vi "sv_Swept Sine Check for Shift Register.vi"(6 "initialize":bool, 8 "error in (no error)":errorcluster, 9 "elapsed time [s]":dbl format="%.2f") -> (0 "error out":errorcluster, 1 "dup elapsed time [s]":dbl format="%.2f")   [LabVIEW 2017, in "SoundVib_SweptSine.lvlib"]
uses:
  <vilib>/addons/Sound and Vibration/svt_Swept Sine/SoundVib_SweptSine.lvlib
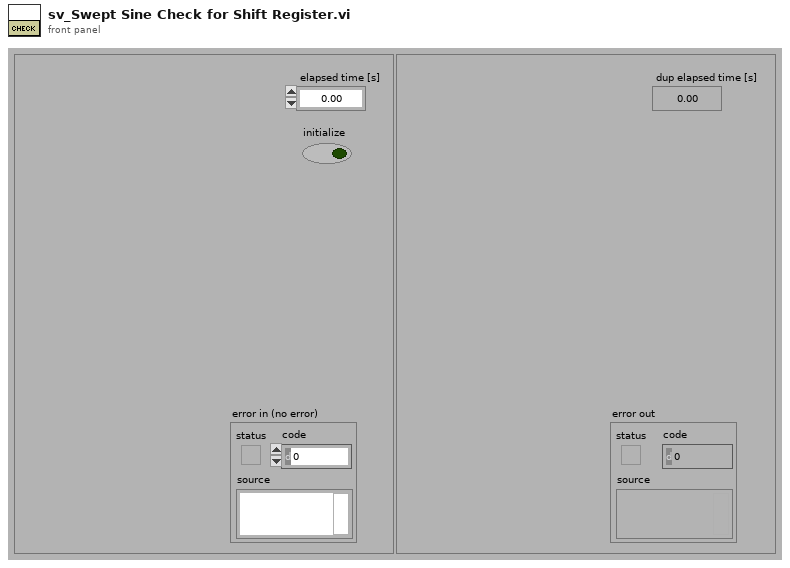
[diagram p1: front panel]
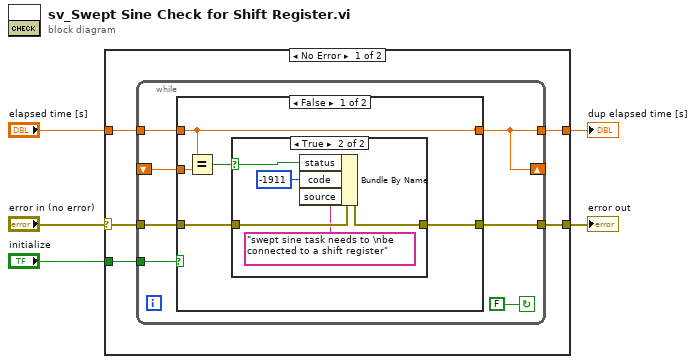
[diagram p0: block diagram]
diagram:
  n1 = case shown="No Error" "error in (no error)" {
    selector: "error in (no error)" -> [w8 w31]
    tunnel: "elapsed time [s]" -> [w10 w32]
    tunnel: "initialize" -> [w9 _]
    tunnel: [w7 w31] -> w3
    tunnel: [w6 w32] -> w2
    frame No Error {
      n2 = while {
        shift-right: [w11] -> _
        shift-left: _ -> [w12]
        tunnel: w10 -> [w13]
        tunnel: w9 -> [w16]
        tunnel: w8 -> [w15]
        tunnel: [w14] -> w7
        tunnel: [w11] -> w6
        stop <- FALSE continue-if-true
        n3 = case shown="False" w16 {
          tunnel: w15 -> [w19 w30]
          tunnel: [w18 w30] -> w14
          tunnel: w13 -> [w22 w29]
          tunnel: [w22 w29] -> w11
          tunnel: w12 -> [w21 _]
          frame False {
            n4 = Equal?(x=w22, y=w21) -> (x = y?=w20:bool)
            n5 = case shown="True" w20 {
              selector: w20 -> [_ w26]
              tunnel: w19 -> [w23 w28]
              tunnel: [w23 w27] -> w18
              frame False {
              }
              frame True {
                n6 = Bundle By Name(cluster=w28, "status"=w26, "code"=-1911, "source"="swept sine task needs to \nbe connected to a shift register") -> (w27:errorcluster)
              }
            }
          }
          frame True {
          }
        }
      }
    }
    frame Error {
    }
  }
  "dup elapsed time [s]" <- w2
  "error out" <- w3
